vi "sensor tray vacuum control.vi"() -> ()   [LabVIEW 2016]
uses:
  Classes/Controllers/I-O/Copy of NI-DAQ Folder/NI-DAQ.lvclass
  Classes/Controllers/I-O/Copy of I-O Folder/I-O.lvclass
  D:/INTT/V1/Classes/Controllers/I-O/Copy of I-O Folder/I-O.lvclass
panel:
  out "Numeric":i32
  in  "Release B":bool
  in  "Release A":bool
  in  "Stop":bool
  in  "TrayVaccum":bool
  in  "Values":bool[](array[boolean])=[FALSE, FALSE]
  out "Vacuum ON?":bool[](array[boolean])
  in  "sample vacuum":i32[](array[numeric])=[13, 19]
  # "Sensor B short"
  # "Sensor A long"
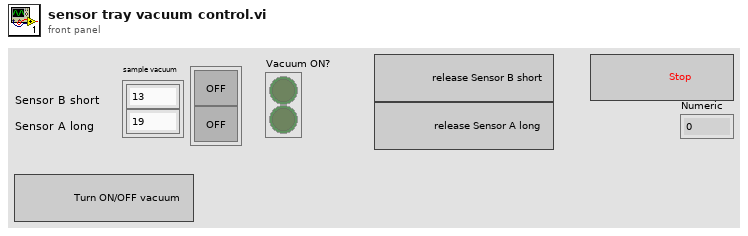
[diagram p1: front panel]
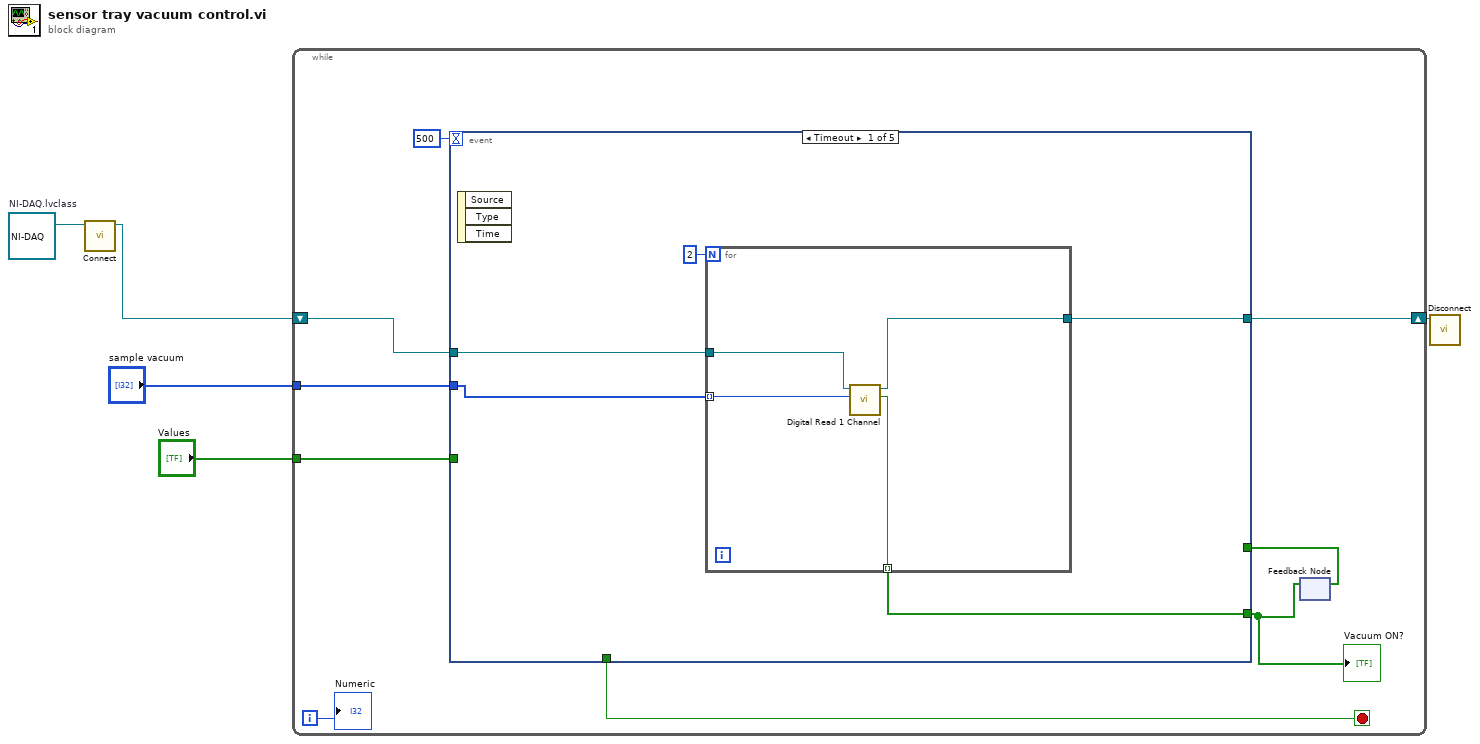
[diagram p0: block diagram]
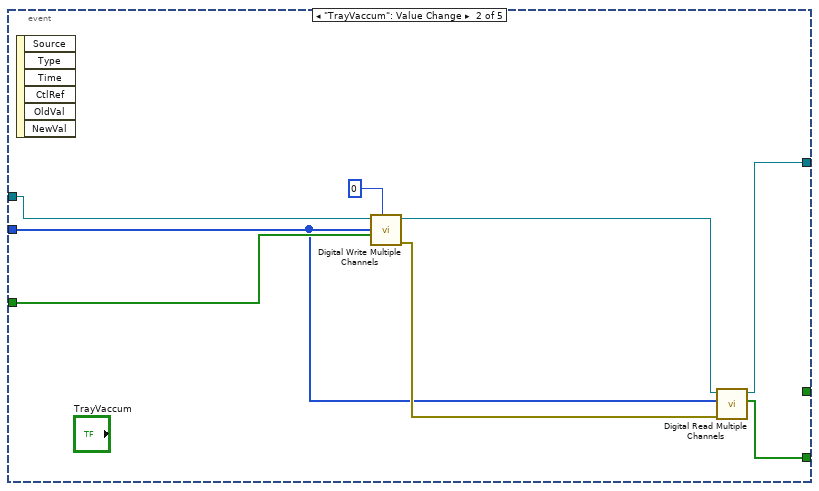
[diagram p2: hidden frame]
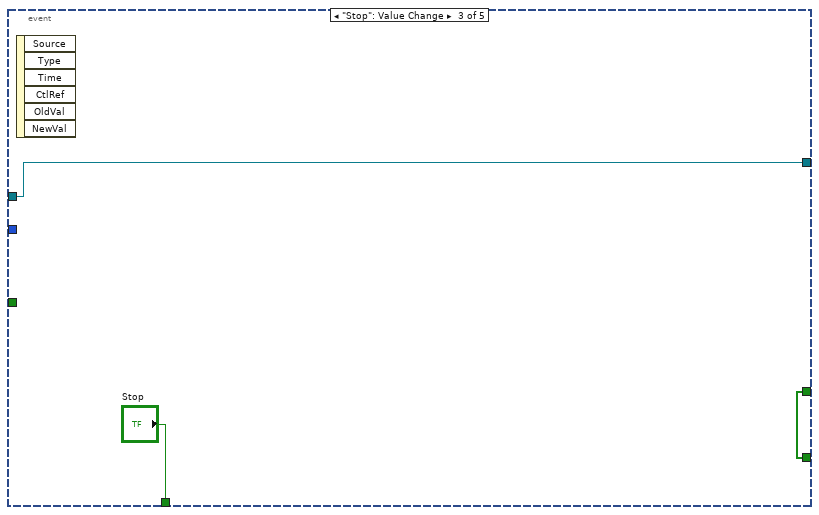
[diagram p3: hidden frame]
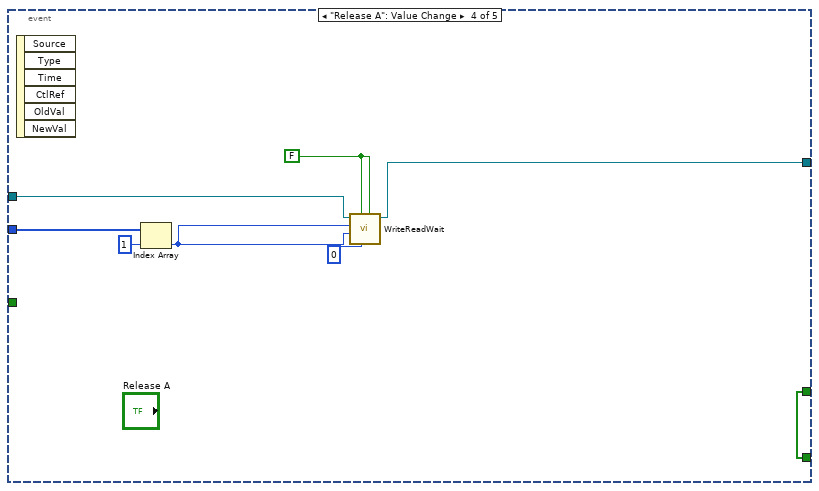
[diagram p4: hidden frame]
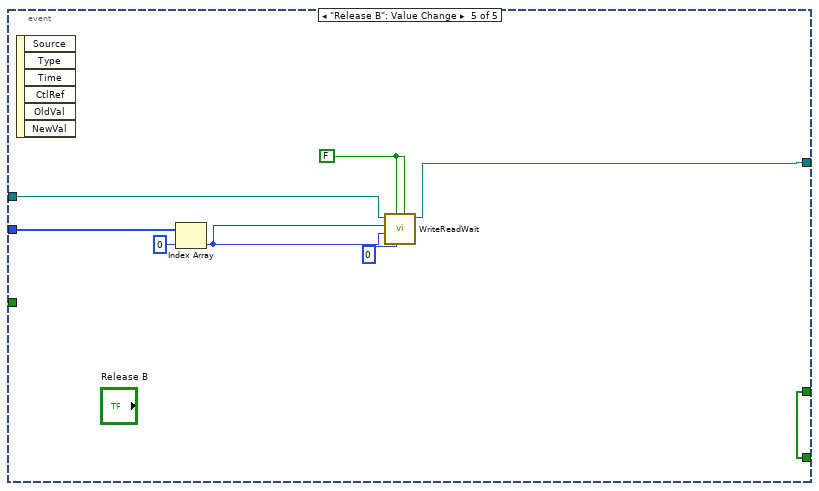
[diagram p5: hidden frame]
diagram:
  w5 = refnum<class "NI-DAQ.lvclass"> refnum  # NI-DAQ.lvclass
  n1 = call-dynamic "Connect.vi"("NI-DAQ in"=w5) -> ("NI-DAQ out"=w3:refnum<class "NI-DAQ.lvclass">)  [unwired: 9 in, 1 out]
  n2 = while {
    tunnel: "sample vacuum" -> [w14]
    shift-right: [w12] -> w2
    shift-left: w3 -> [w13]
    tunnel: "Values" -> [w11]
    i -> [w8]
    stop <- w10 stop-if-true
    n3 = feedback #1() -> (w6:bool[])  [unwired: 1 in]
    n4 = event shown="[0] Timeout" {
      selector: _ -> [_ _ _ _ _]
      dyn-events: _ -> [_ _ _ _ _]
      timeout: 500 -> [_ _ _ _ _]
      tunnel: w14 -> [w17 w24 _ w40 w45]
      tunnel: w13 -> [w18 w29 w34 w41 w48]
      tunnel: [w16 w31 w34 w37 w47] -> w12
      tunnel: w11 -> [_ w27 _ _ _]
      tunnel: [w15 w30 w32 w35 w43] -> w7
      tunnel: [_ _ "Stop" _ _] -> w10
      tunnel: w6 -> [_ _ w32 w35 w43]
      event Timeout {
        n5 = event-data() -> ()  [unwired: 1 in, 3 out]
        n6 = for {
          N: 2 -> [_]
          tunnel: w18 -> [w23]
          tunnel: w17 -> [w22] mode=indexing
          tunnel: [w21] -> w16
          tunnel: [w20] -> w15 mode=indexing
          n7 = call-dynamic "Digital Read 1 Channel.vi"("Read"=w22, "NI-DAQ in"=w23) -> ("Value"=w20:bool, "NI-DAQ out"=w21:refnum<class "NI-DAQ.lvclass">)  [unwired: 7 in, 1 out]
        }
      }
      event "TrayVaccum": Value Change {
        n8 = event-data() -> ()  [unwired: 1 in, 6 out]
        n9 = call-dynamic "Digital Write Multiple Channels.vi"("DAQ Module"=0, "Values"=w27, "Indices"=w24, "NI-DAQ in"=w29) -> ("error out"=w25:errorcluster, "NI-DAQ out"=w26:refnum<class "NI-DAQ.lvclass">)  [unwired: 6 in]
        n10 = call-dynamic "Digital Read Multiple Channels.vi"("error in (no error)"=w25, "Array"=w24, "NI-DAQ in"=w26) -> ("subarray"=w30:bool[], "NI-DAQ out"=w31:refnum<class "NI-DAQ.lvclass">)  [unwired: 6 in, 1 out]
      }
      event "Stop": Value Change {
        n11 = event-data() -> ()  [unwired: 1 in, 6 out]
      }
      event "Release A": Value Change {
        w42 = FALSE
        n12 = event-data() -> ()  [unwired: 1 in, 6 out]
        n13 = Index Array(array=w40, index=1) -> (element=w38:i32)
        n14 = call "WriteReadWait.vi"("Read Value"=w42, 6:0 ("DAQ Module"), "Write Value"=w42, "Read"=w38, "Write"=w38, "I-O in"=w41) -> ("I-O out"=w37:refnum<class "NI-DAQ.lvclass">)  [unwired: 4 in, 1 out]
      }
      event "Release B": Value Change {
        w49 = FALSE
        n15 = event-data() -> ()  [unwired: 1 in, 6 out]
        n16 = Index Array(array=w45, index=0) -> (element=w46:i32)
        n17 = call "WriteReadWait.vi"("Read Value"=w49, 6:0 ("DAQ Module"), "Write Value"=w49, "Read"=w46, "Write"=w46, "I-O in"=w48) -> ("I-O out"=w47:refnum<class "NI-DAQ.lvclass">)  [unwired: 4 in, 1 out]
      }
    }
    "Vacuum ON?" <- w7
    n18 = feedback-in #1(w7) -> ()
    "Numeric" <- w8
  }
  n19 = call-dynamic "Disconnect.vi"("I-O in"=w2) -> ()  [unwired: 9 in, 1 out]
